vi "Send Set most in front and shift.vi"(8 "error in (no error)":errorcluster, 10 "top left point":cluster{"x":i16, "y":i16}, 11 "Message Enqueuer in":refnum<class "Message Enqueuer.lvclass">) -> (0 "error out":errorcluster)   [LabVIEW 2020, in "ViewableActor.lvlib"]
uses:
  ViewableActor.lvlib
  <vilib>/ActorFramework/Message Enqueuer/Message Enqueuer.lvclass
  Set IsFrontMost Msg/Set IsFrontMost Msg.lvclass/Set IsFrontMost Msg.ctl
  <vilib>/ActorFramework/Message Enqueuer/Message Enqueuer.lvclass/Message Enqueuer.ctl
  Shift Window Msg/Shift Window Msg.lvclass/Shift Window Msg.ctl
  <vilib>/ActorFramework/Message Enqueuer/Enqueue.vi
  Set IsFrontMost Msg/Set IsFrontMost Msg.lvclass
  C:/Program Files (x86)/National Instruments/LabVIEW 2020/vi.lib/ActorFramework/Message/Message.lvclass
  Shift Window Msg/Shift Window Msg.lvclass
  <vilib>/ActorFramework/Message Priority Queue/Priority Enqueue.vi
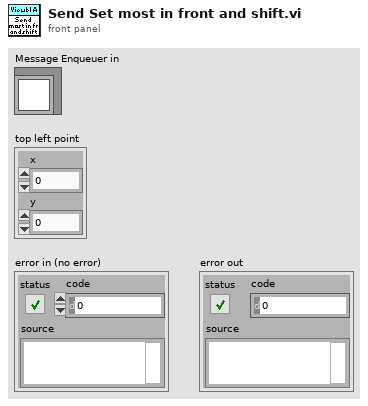
[diagram p1: front panel]
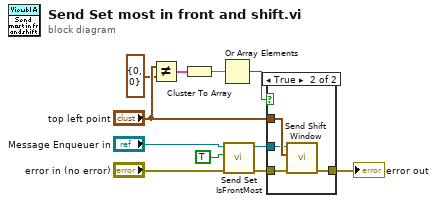
[diagram p0: block diagram]
diagram:
  n1 = Not Equal?(x="top left point", y=cluster{"x":i16, "y":i16} {"x"=0, "y"=0} ("x")) -> (x != y?=w4:cluster{"x":bool, "y":bool})
  n2 = Cluster To Array(cluster=w4) -> (array=w5:bool[])
  n3 = Or Array Elements(Boolean array=w5) -> (logical OR=w7:bool)
  n4 = call "Send Set IsFrontMost.vi"("error in (no error)"="error in (no error)", "IsFrontMost"=TRUE, "Message Enqueuer"="Message Enqueuer in") -> ("error out"=w2:errorcluster, "Message Enqueuer out"=w6:refnum<class "Message Enqueuer.lvclass">)  [unwired: 7 in]
  n5 = case shown="True" w7 {
    tunnel: w2 -> [w12 w15]
    tunnel: [w12 w14] -> w8
    tunnel: w6 -> [_ w13]
    tunnel: "top left point" -> [_ w16]
    frame False {
    }
    frame True {
      n6 = call "Send Shift Window.vi"("error in (no error)"=w15, "top left point"=w16, "Message Enqueuer"=w13) -> ("error out"=w14:errorcluster)  [unwired: 7 in, 1 out]
    }
  }
  "error out" <- w8
